vi "GA_INJECT_PLATE.vi"(8 "Error IN":errorcluster, 9 "Wells to Inject":T1[](array[typedef])=[{"Column"=enum."1", "Row"=enum."A"}, {"Column"=enum."1", "Row"=enum."E"}, {"Column"=enum."4", "Row"=enum."F"}, {"Column"=enum."11", "Row"=enum."H"}, {"Column"=enum."2", "Row"=enum."C"}], 10 "Loader Settings":T4={"Sample Flow Rate (uL/s)"=10.0, "Sample Volume (uL)"=80.0, "Mixing Volume (uL)"=200, "Mixing Speed (uL/s)"=1, "Mix#"=5, "Wash Volume (uL)"=100, "INJECTION_MODE"=enum."HT"} {"Sample Volume (uL)" min=2.0 max=200.0 step=0.5; "Mixing Volume (uL)" min=5 max=100 step=5; "Mixing Speed (uL/s)" min=25 max=250 step=5; "Sample Flow Rate (uL/s)" min=0.5 max=3.0 step=0.5 format="%_2f"; "Mix#" min=0 max=5 step=1; "Wash Volume (uL)" min=200 max=800 step=20}, 11 "VISA resource IN":refnum<visa-resource-name>="HTS") -> (0 "errorOUT":errorcluster, 3 "VISA resource OUT":refnum<visa-resource-name>)   [LabVIEW 2009]
uses:
  HTS_LOADER_SETTINGS.ctl
  HTS_INJECTION_MODE.ctl
  HTS_WELL.ctl
  HTS_COLUMN.ctl
  HTS_ROW.ctl
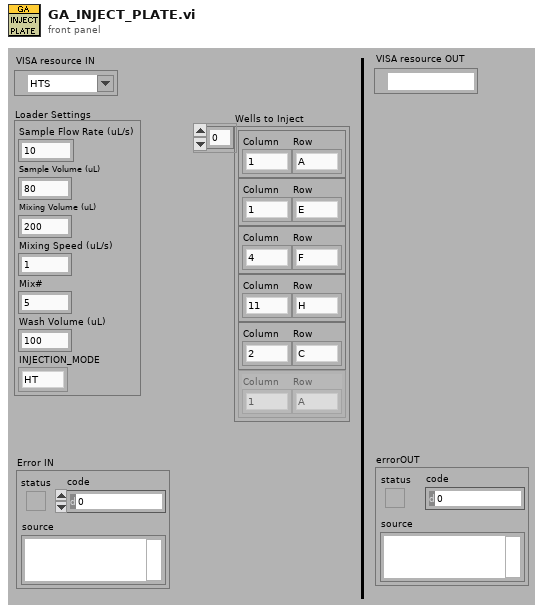
[diagram p1: front panel]
types:
  T1 = typedef "HTS_WELL.ctl" = cluster{"Column":T2, "Row":T3}
  T2 = typedef "HTS_COLUMN.ctl" = enum16{"1", "2", "3", "4", "5", "6", "7", "8", "9", "10", "11", "12"}
  T3 = typedef "HTS_ROW.ctl" = enum16{"A", "B", "C", "D", "E", "F", "G", "H"}
  T4 = typedef "HTS_LOADER_SETTINGS.ctl" = cluster{"Sample Flow Rate (uL/s)":dbl, "Sample Volume (uL)":dbl, "Mixing Volume (uL)":i32, "Mixing Speed (uL/s)":i32, "Mix#":i32, "Wash Volume (uL)":i32, "INJECTION_MODE":T5}
  T5 = typedef "HTS_INJECTION_MODE.ctl" = enum16{"STD", "HT"}
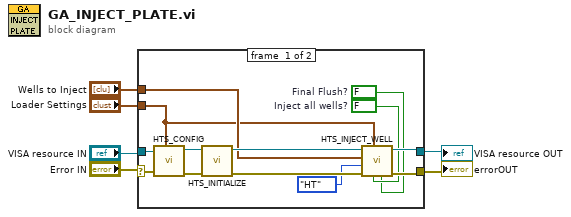
[diagram p0: block diagram]
diagram:
  n1 = case shown="No Error" "Error IN" {
    selector: "Error IN" -> [w18 w20]
    tunnel: "Loader Settings" -> [w8 _]
    tunnel: "VISA resource IN" -> [w19 w21]
    tunnel: "Wells to Inject" -> [w9 _]
    tunnel: [w14 w20] -> w2
    tunnel: [w12 w21] -> w1
    frame #0 {
      w10 = FALSE  # Final Flush?
      w11 = FALSE  # Inject all wells?
      n2 = call "HTS_CONFIG.vi"("Loader Settings"=w8, "error IO"=w18, "VISA resource IN"=w19) -> ("Error OUT"=w17:errorcluster, "VISA resource OUT"=w16:refnum<visa-resource-name>)  [unwired: 5 out]
      n3 = call "HTS_INITIALIZE.vi"("Error IN"=w17, "VISA resource IN"=w16) -> ("Error OUT"=w15:errorcluster, "VISA resource OUT"=w13:refnum<visa-resource-name>)  [unwired: 6 out]
      n4 = call "HTS_INJECT_WELL.vi"("Final Flush?"=w10, "Inject all wells?"=w11, "Loader Settings"=w8, "Error IN"=w15, "INJECTION_MODE"=HTS_INJECTION_MODE."HT", "Wells to Inject"=w9, "VISA resource IN"=w13) -> ("Error OUT"=w14:errorcluster, "VISA resource OUT"=w12:refnum<visa-resource-name>)  [unwired: 2 in, 1 out]
    }
    frame #1 {
    }
  }
  "errorOUT" <- w2
  "VISA resource OUT" <- w1
